vi "TestOderProtokollUi.vi"(11 "Data in":T1={"Report.lvclass"=refnum, "Norm"="", "last State"=enum."Initialize", "Norm ID"=0, "parameter"=[], "EMTestCWS500N.lvclass"=refnum, "CEG4500.lvclass"=refnum, "Tektronix RSA5106A.lvclass"=refnum, "erfolgreich"=FALSE, "log"="", "Kommentar"="", "Device Enum"=enum."emTestCWS500N", "Test Enum"=enum."HF-Felder", "debug"=FALSE, "tab"=enum."Hauptmenü", "ESD Pistol.lvclass"=refnum, "SubPnl Refnum"=refnum}) -> (2 "TestMitGerät out":bool, 3 "Data out":T1={"Report.lvclass"=refnum, "Norm"="", "last State"=enum."Initialize", "Norm ID"=0, "parameter"=[], "EMTestCWS500N.lvclass"=refnum, "CEG4500.lvclass"=refnum, "Tektronix RSA5106A.lvclass"=refnum, "erfolgreich"=FALSE, "log"="", "Kommentar"="", "Device Enum"=enum."emTestCWS500N", "Test Enum"=enum."HF-Felder", "debug"=FALSE, "tab"=enum."Hauptmenü", "ESD Pistol.lvclass"=refnum, "SubPnl Refnum"=refnum})   [LabVIEW 2013]
uses:
  Main/controls/Data.ctl
  classes/Datastructure/Report/Report.lvclass
  classes/Devices/emTestCWS500N/EMTestCWS500N.lvclass
  classes/Devices/CEG4500/CEG4500.lvclass
  classes/Devices/Tektronix RSA5106A/Tektronix RSA5106A.lvclass
  ESD Pistol.lvclass
  Main/controls/State.ctl
  classes/Devices/DeviceInterface/Devices.ctl
  classes/Tests/TestInterface/Tests.ctl
  Tabs.ctl
  classes/Tests/TestInterface/TestInterface.lvclass
  classes/Devices/DeviceInterface/DeviceInterface.lvclass
  classes/Tests/Stoeraussendung/Stoeraussendung.lvclass
  classes/Tests/Burst/Burst.lvclass
  classes/Tests/Surge/Surge.lvclass
  classes/Tests/Spannungseinbruch/Spannungseinbruch.lvclass
  classes/Tests/HF-Felder/HF-Felder.lvclass
  classes/Tests/ESD/ESD.lvclass
panel:
  out "error out":errorcluster
  in  "error in":errorcluster
  in  "TestOhneGerät":bool
  in  "TestMitGerät":bool
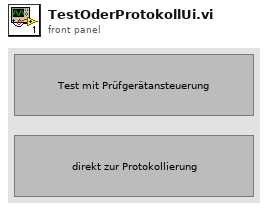
[diagram p1: front panel]
types:
  T1 = typedef "Data.ctl" = cluster{"Report.lvclass":refnum<class "Report.lvclass">, "Norm":string, "last State":T2, "Norm ID":i32, "parameter":string[][], "EMTestCWS500N.lvclass":refnum<class "EMTestCWS500N.lvclass">, "CEG4500.lvclass":refnum<class "CEG4500.lvclass">, "Tektronix RSA5106A.lvclass":refnum<class "Tektronix RSA5106A.lvclass">, "erfolgreich":bool, "log":string, "Kommentar":string, "Device Enum":T3, "Test Enum":T4, "debug":bool, "tab":T5, "ESD Pistol.lvclass":refnum<class "ESD Pistol.lvclass">, "SubPnl Refnum":refnum<vi>}
  T2 = typedef "State.ctl" = enum16{"create Pdf", "load Report", "save Report", "do Test", "CDN Kalibrierung", "enter Report Parameters", "new Test", "Protokoll", "read Tree", "update Tree", "Fehler", "Initialize", "Wait for Event", "Exit"}
  T3 = typedef "Devices.ctl" = enum16{"unbekannt", "ESD Pistol", "Tektronix RSA5106A", "emTestCWS500N", "CEG-4500"}
  T4 = typedef "Tests.ctl" = enum16{"unbekannt", "Störaussendung", "Burst", "ESD", "Surge", "Spannungseinbruch", "HF-Felder"}
  T5 = typedef "Tabs.ctl" = enum32{"Hauptmenü", "Prüfbericht", "Einstellungen"}
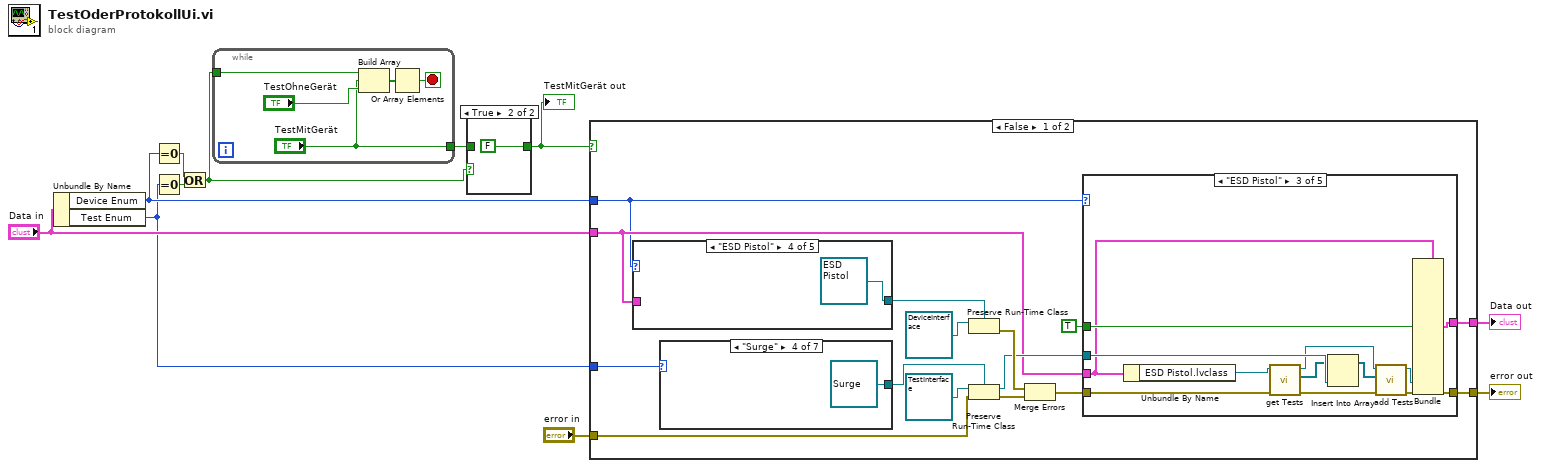
[diagram p0: block diagram]
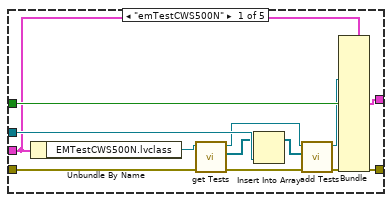
[diagram p2: hidden frame]
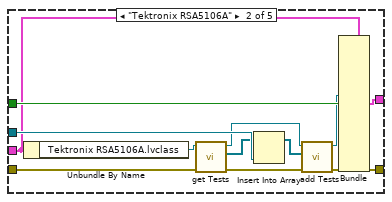
[diagram p3: hidden frame]
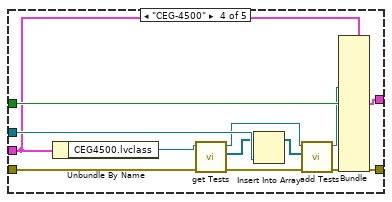
[diagram p4: hidden frame]
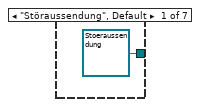
[diagram p6: hidden frame]
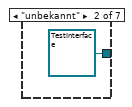
[diagram p7: hidden frame]
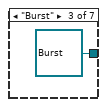
[diagram p8: hidden frame]
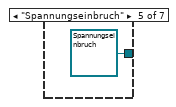
[diagram p9: hidden frame]
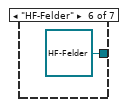
[diagram p10: hidden frame]
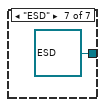
[diagram p11: hidden frame]
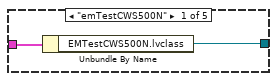
[diagram p12: hidden frame]
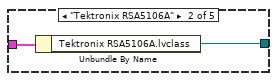
[diagram p13: hidden frame]
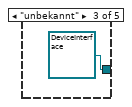
[diagram p14: hidden frame]
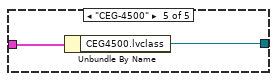
[diagram p15: hidden frame]
diagram:
  n1 = Unbundle By Name("Data in") -> ("Device Enum"=w3:T3, "Test Enum"=w2:T4)
  n2 = Equal To 0?(x=w3) -> (x = 0?=w11:bool)
  n3 = Equal To 0?(x=w2) -> (x = 0?=w10:bool)
  n4 = Or(x=w11, y=w10) -> (x .or. y?=w8:bool)
  n5 = while {
    tunnel: ["TestMitGerät"] -> w9
    tunnel: w8 -> [w14]
    stop <- w13 stop-if-true
    n6 = Build Array(w14, "TestMitGerät", "TestOhneGerät") -> (w12:bool[])
    n7 = Or Array Elements(Boolean array=w12) -> (logical OR=w13:bool)
  }
  n8 = case shown="True" w8 {
    tunnel: w9 -> [w17 _]
    tunnel: [w17 FALSE] -> w4
    frame False {
    }
    frame True {
    }
  }
  "TestMitGerät out" <- w4
  n9 = case shown="False" w4 {
    tunnel: w2 -> [w32 _]
    tunnel: "Data in" -> [w24 w100]
    tunnel: w3 -> [w23 _]
    tunnel: [w21 w100] -> w6
    tunnel: [w20 w99] -> w5
    tunnel: "error in" -> [w19 w99]
    frame False {
      n10 = case shown="\"ESD Pistol\"" w23 {
        tunnel: [w91 w93 refnum<class "DeviceInterface.lvclass"> refnum ("Tektronix RSA5106A.lvclass") refnum<class "ESD Pistol.lvclass"> refnum ("ESD Pistol.lvclass") w97] -> w33
        tunnel: w24 -> [w92 w94 _ _ w98]
        frame "emTestCWS500N" {
          n11 = Unbundle By Name(w92) -> ("EMTestCWS500N.lvclass"=w91:refnum<class "EMTestCWS500N.lvclass">)
        }
        frame "Tektronix RSA5106A" {
          n12 = Unbundle By Name(w94) -> ("Tektronix RSA5106A.lvclass"=w93:refnum<class "Tektronix RSA5106A.lvclass">)
        }
        frame "unbekannt" {
        }
        frame "ESD Pistol" {
        }
        frame "CEG-4500" {
          n13 = Unbundle By Name(w98) -> ("CEG4500.lvclass"=w97:refnum<class "CEG4500.lvclass">)
        }
      }
      n14 = case shown="\"Surge\"" w32 {
        tunnel: [refnum<class "Stoeraussendung.lvclass"> refnum ("Störaussendung.lvclass") refnum<class "TestInterface.lvclass"> refnum ("Burst.lvclass") refnum<class "Burst.lvclass"> refnum ("Burst.lvclass") refnum<class "Surge.lvclass"> refnum ("Surge.lvclass") refnum<class "Spannungseinbruch.lvclass"> refnum ("Spannungseinbruch.lvclass") refnum<class "HF-Felder.lvclass"> refnum ("HF-Felder.lvclass") refnum<class "ESD.lvclass"> refnum ("ESD.lvclass")] -> w29
        frame "Störaussendung", Default {
        }
        frame "unbekannt" {
        }
        frame "Burst" {
        }
        frame "Surge" {
        }
        frame "Spannungseinbruch" {
        }
        frame "HF-Felder" {
        }
        frame "ESD" {
        }
      }
      n15 = Preserve Run-Time Class(object in=refnum<class "DeviceInterface.lvclass"> refnum ("DeviceInterface.lvclass"), 2:w33) -> (error out=w31:errorcluster)  [unwired: 1 in, 1 out]
      n16 = Preserve Run-Time Class(object in=refnum<class "TestInterface.lvclass"> refnum ("TestInterface.lvclass"), error in=w19, 2:w29) -> (object out=w26:refnum<class "TestInterface.lvclass">, error out=w30:errorcluster)
      n17 = Merge Errors(w31, w30) -> (w25:errorcluster)
      n18 = case shown="\"ESD Pistol\"" w23 {
        tunnel: TRUE ("erfolgreich") -> [w45 w57 w69 w81 _]
        tunnel: w26 -> [w44 w56 w68 w80 _]
        tunnel: w25 -> [w43 w55 w67 w79 w83]
        tunnel: [w42 w54 w66 w78 w83] -> w20
        tunnel: [w40 w52 w65 w77 w82] -> w21
        tunnel: w24 -> [w39 w51 w64 w75 w82]
        frame "emTestCWS500N" {
          n19 = Unbundle By Name(w39) -> ("EMTestCWS500N.lvclass"=w38:refnum<class "EMTestCWS500N.lvclass">)
          n20 = call-dynamic "get Tests.vi"("error in (no error)"=w43, "DeviceInterface (Eingang)"=w38) -> ("error out"=w34:errorcluster, "Tests"=w37:refnum<class "TestInterface.lvclass">[], "DeviceInterface (Ausgang)"=w35:refnum<class "EMTestCWS500N.lvclass">)  [unwired: 7 in]
          n21 = Insert Into Array(array=w37, new element=w44) -> (w36:refnum<class "TestInterface.lvclass">[])  [unwired: 1 in]
          n22 = call-dynamic "add Tests.vi"("error in (no error)"=w34, "Tests"=w36, "DeviceInterface (Eingang)"=w35) -> ("error out"=w42:errorcluster, "DeviceInterface (Ausgang)"=w41:refnum<class "EMTestCWS500N.lvclass">)  [unwired: 7 in]
          n23 = Bundle(cluster=w39, "EMTestCWS500N.lvclass"=w41, "erfolgreich"=w45) -> (w40:T1)  [unwired: 15 in]
        }
        frame "Tektronix RSA5106A" {
          n24 = Unbundle By Name(w51) -> ("Tektronix RSA5106A.lvclass"=w50:refnum<class "Tektronix RSA5106A.lvclass">)
          n25 = call-dynamic "get Tests.vi"("error in (no error)"=w55, "DeviceInterface (Eingang)"=w50) -> ("error out"=w46:errorcluster, "Tests"=w49:refnum<class "TestInterface.lvclass">[], "DeviceInterface (Ausgang)"=w47:refnum<class "Tektronix RSA5106A.lvclass">)  [unwired: 7 in]
          n26 = Insert Into Array(array=w49, new element=w56) -> (w48:refnum<class "TestInterface.lvclass">[])  [unwired: 1 in]
          n27 = call-dynamic "add Tests.vi"("error in (no error)"=w46, "Tests"=w48, "DeviceInterface (Eingang)"=w47) -> ("error out"=w54:errorcluster, "DeviceInterface (Ausgang)"=w53:refnum<class "Tektronix RSA5106A.lvclass">)  [unwired: 7 in]
          n28 = Bundle(cluster=w51, "Tektronix RSA5106A.lvclass"=w53, "erfolgreich"=w57) -> (w52:T1)  [unwired: 15 in]
        }
        frame "ESD Pistol" {
          n29 = Unbundle By Name(w64) -> ("ESD Pistol.lvclass"=w63:refnum<class "ESD Pistol.lvclass">)
          n30 = call-dynamic "get Tests.vi"("error in (no error)"=w67, "DeviceInterface (Eingang)"=w63) -> ("error out"=w59:errorcluster, "Tests"=w62:refnum<class "TestInterface.lvclass">[], "DeviceInterface (Ausgang)"=w60:refnum<class "ESD Pistol.lvclass">)  [unwired: 7 in]
          n31 = Insert Into Array(array=w62, new element=w68) -> (w61:refnum<class "TestInterface.lvclass">[])  [unwired: 1 in]
          n32 = call-dynamic "add Tests.vi"("error in (no error)"=w59, "Tests"=w61, "DeviceInterface (Eingang)"=w60) -> ("error out"=w66:errorcluster, "DeviceInterface (Ausgang)"=w58:refnum<class "ESD Pistol.lvclass">)  [unwired: 7 in]
          n33 = Bundle(cluster=w64, "erfolgreich"=w69, "ESD Pistol.lvclass"=w58) -> (w65:T1)  [unwired: 15 in]
        }
        frame "CEG-4500" {
          n34 = Unbundle By Name(w75) -> ("CEG4500.lvclass"=w74:refnum<class "CEG4500.lvclass">)
          n35 = call-dynamic "get Tests.vi"("error in (no error)"=w79, "DeviceInterface (Eingang)"=w74) -> ("error out"=w70:errorcluster, "Tests"=w73:refnum<class "TestInterface.lvclass">[], "DeviceInterface (Ausgang)"=w71:refnum<class "CEG4500.lvclass">)  [unwired: 7 in]
          n36 = Insert Into Array(array=w73, new element=w80) -> (w72:refnum<class "TestInterface.lvclass">[])  [unwired: 1 in]
          n37 = call-dynamic "add Tests.vi"("error in (no error)"=w70, "Tests"=w72, "DeviceInterface (Eingang)"=w71) -> ("error out"=w78:errorcluster, "DeviceInterface (Ausgang)"=w76:refnum<class "CEG4500.lvclass">)  [unwired: 7 in]
          n38 = Bundle(cluster=w75, "CEG4500.lvclass"=w76, "erfolgreich"=w81) -> (w77:T1)  [unwired: 15 in]
        }
        frame "unbekannt" {
        }
      }
    }
    frame True {
    }
  }
  "Data out" <- w6
  "error out" <- w5
